vi "getWriteFile.vi"(0 "refnum in":refnum<file>, 1 "from (0:start)":enum16{"start", "end", "current"}(ring), 2 "offset (in bytes) (0)":i64, 3 "error in":errorcluster, 4 "Data":string[][](array[string])) -> (5 "refnum out":refnum<file>, 6 "position after write(bytes)":i32, 7 "error out":errorcluster)   [LabVIEW 2013]
uses:
  <vilib>/Utility/file.llb/Write To Spreadsheet File (string).vi
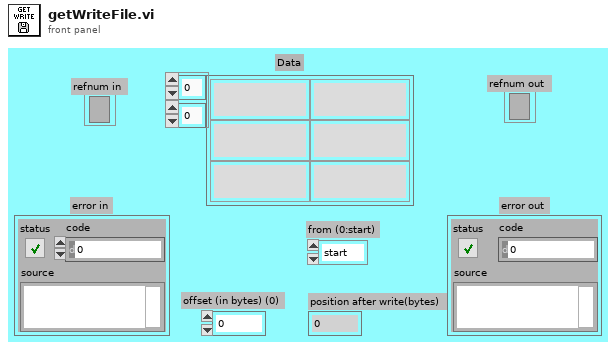
[diagram p1: front panel]
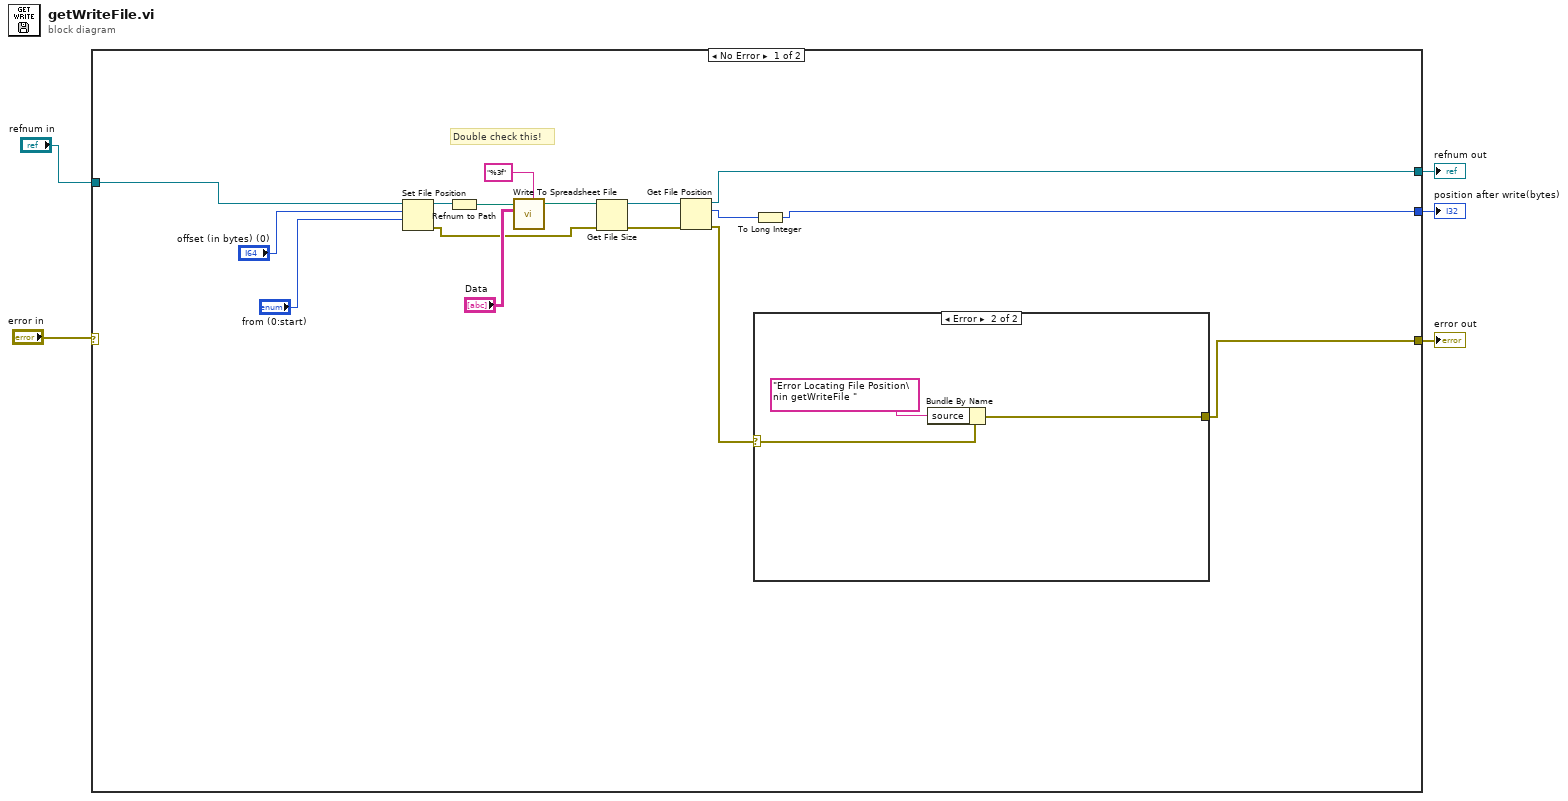
[diagram p0: block diagram]
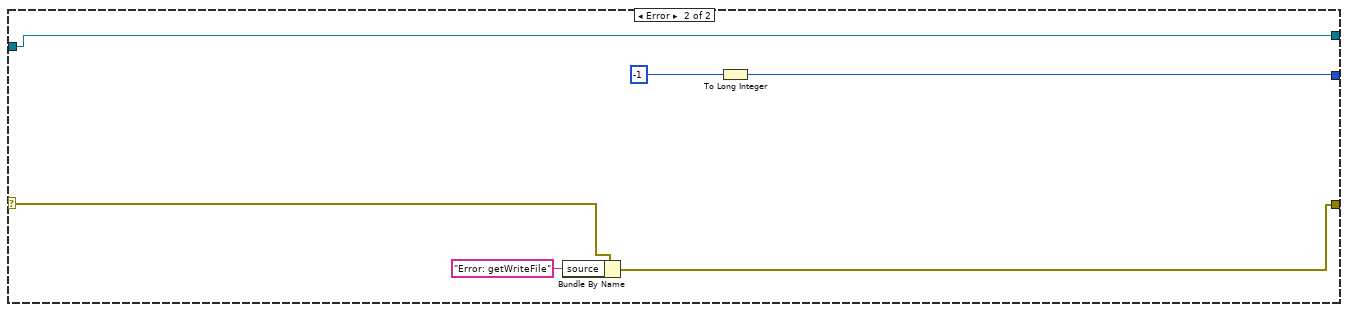
[diagram p3: hidden frame]
diagram:
  n1 = case shown="No Error" "error in" {
    selector: "error in" -> [_ w28]
    tunnel: "refnum in" -> [w18 w31]
    tunnel: [w16 w26] -> w1
    tunnel: [w15 w29] -> w2
    tunnel: [w11 w31] -> w3
    frame No Error {
      # "Double check this!"
      n2 = Set File Position(offset (in bytes) (0)="offset (in bytes) (0)", refnum=w18, from (0:start)="from (0:start)") -> (refnum out=w14:refnum<file>, error out=w8:errorcluster)  [unwired: 1 in]
      n3 = Refnum to Path(1:w14) -> (0:w13:path)
      n4 = call-poly <vilib>:"Write To Spreadsheet File.vi"("format (%s)"="%3f", "2D data"="Data", "file path (dialog if empty)"=w13) -> ("new file path (Not A Path if cancelled)"=w10:path)  [unwired: 5 in]
      n5 = Get File Size(file=w10, error in=w8) -> (refnum out=w9:refnum<file>, 0:w7:errorcluster)  [unwired: 1 out]
      n6 = Get File Position(4:w7, 7:w9) -> (0:w17:errorcluster, 2:w19:i64, 3:w11:refnum<file>)
      n7 = case shown="Error" w17 {
        selector: w17 -> [w22 w25]
        tunnel: [w22 w23] -> w16
        frame No Error {
        }
        frame Error {
          n8 = Bundle By Name(cluster=w25, "source"="Error Locating File Position\nin getWriteFile ") -> (w23:errorcluster)
        }
      }
      n9 = To Long Integer(number=w19) -> (32bit integer=w15:i32)
    }
    frame Error {
      n10 = Bundle By Name(cluster=w28, "source"="Error: getWriteFile") -> (w26:errorcluster)
      n11 = To Long Integer(number=-1) -> (32bit integer=w29:i32)
    }
  }
  "refnum out" <- w3
  "position after write(bytes)" <- w2
  "error out" <- w1
